vi "Sweep Set.vi"(8 "error in (no error)":errorcluster, 9 "Sweep outfile":path, 10 "addr":i32, 11 "instrument handle":refnum<k15>) -> (0 "error out":errorcluster, 1 "final current (A)":dbl, 2 "final resistance (ohm)":dbl, 3 "instrument handle out":refnum<k15>)   [LabVIEW 2018]
uses:
  <vilib>/Utility/file.llb/Write Delimited Spreadsheet (DBL).vi
panel:
  out "i":i32
  out "PW":i32
  out "BL voltage (V)":dbl
  out "WL voltage (V)":dbl
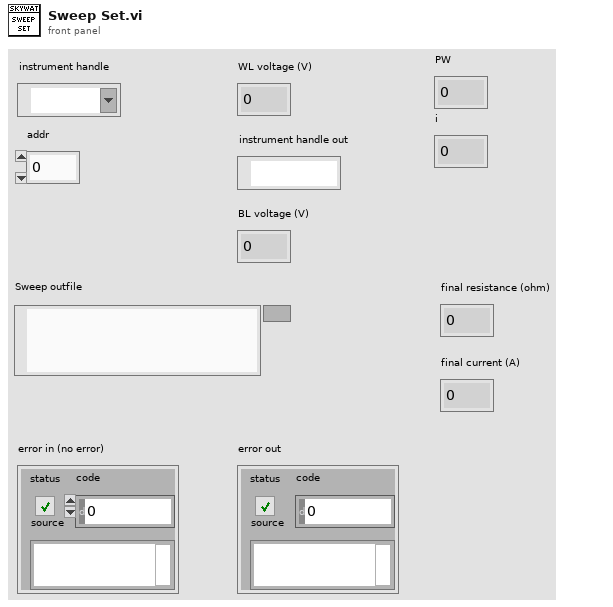
[diagram p1: front panel]
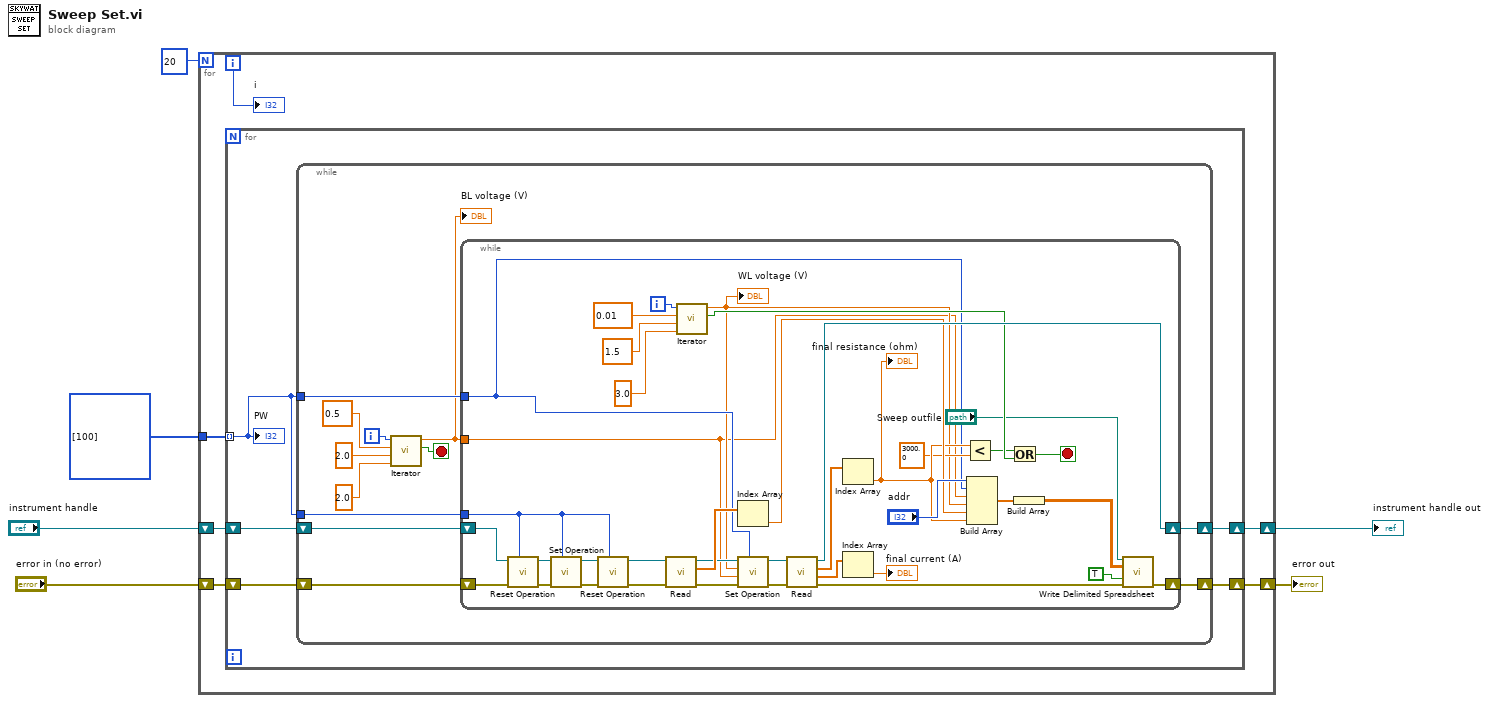
[diagram p0: block diagram]
diagram:
  n1 = for {
    N: 20 -> [_]
    tunnel: i32[] [100] -> [w8]
    shift-right: [w12] -> w6
    shift-left: "instrument handle" -> [w11]
    shift-right: [w9] -> w3
    shift-left: "error in (no error)" -> [w10]
    i -> [w7]
    n2 = for {
      shift-right: [w17] -> w12
      shift-left: w11 -> [w16]
      shift-right: [w14] -> w9
      shift-left: w10 -> [w15]
      tunnel: w8 -> [w13] mode=indexing
      n3 = while {
        shift-right: [w26] -> w17
        shift-left: w16 -> [w19]
        shift-right: [w25] -> w14
        shift-left: w15 -> [w18]
        tunnel: w13 -> [w23]
        tunnel: w13 -> [w20]
        i -> [w27]
        stop <- w22 stop-if-true
        n4 = call "Iterator.vi"("Final Value"=2.0 ("y"), "Initial Value"=2.0 ("y"), "Step"=0.5 ("x"), "i"=w27) -> ("End Loop"=w22:bool, "Current Value"=w21:dbl)  [unwired: 6 in]
        "BL voltage (V)" <- w21
        n5 = while {
          shift-right: [w57] -> w26
          shift-left: w19 -> [w37]
          shift-right: [w60] -> w25
          shift-left: w18 -> [w34]
          tunnel: w21 -> [w39]
          tunnel: w23 -> [w42]
          tunnel: w20 -> [w38]
          i -> [w67]
          stop <- w51 stop-if-true
          n6 = call "Reset Operation.vi"("PW"=w38, "error in (no error)"=w34, "instrument handle"=w37) -> ("error out"=w33:errorcluster, "instrument handle out"=w32:refnum<k15>)  [unwired: 7 in]
          n7 = call "Set Operation.vi"("PW"=w38, "error in (no error)"=w33, "instrument handle"=w32) -> ("error out"=w31:errorcluster, "instrument handle out"=w30:refnum<k15>)  [unwired: 7 in]
          n8 = call "Reset Operation.vi"("PW"=w38, "error in (no error)"=w31, "instrument handle"=w30) -> ("error out"=w35:errorcluster, "instrument handle out"=w36:refnum<k15>)  [unwired: 7 in]
          n9 = call "Read.vi"("error in (no error)"=w35, "instrument handle"=w36) -> ("error out"=w45:errorcluster, "resistances (ohm)"=w53:dbl[], "instrument handle out"=w46:refnum<k15>)  [unwired: 6 in, 1 out]
          n10 = call "Iterator.vi"("Final Value"=3.0 ("y"), "Initial Value"=1.5 ("y"), "Step"=0.01 ("x"), "i"=w67) -> ("End Loop"=w50:bool, "Current Value"=w40:dbl)  [unwired: 6 in]
          "WL voltage (V)" <- w40
          n11 = Index Array(array=w53) -> (element=w52:dbl)  [unwired: 1 in]
          n12 = call "Set Operation.vi"("PW"=w42, "error in (no error)"=w45, "BLV"=w39, "WLV"=w40, "instrument handle"=w46) -> ("error out"=w44:errorcluster, "instrument handle out"=w43:refnum<k15>)  [unwired: 5 in]
          n13 = call "Read.vi"("error in (no error)"=w44, "instrument handle"=w43) -> ("error out"=w58:errorcluster, "currents (A)"=w55:dbl[], "resistances (ohm)"=w56:dbl[], "instrument handle out"=w57:refnum<k15>)  [unwired: 6 in]
          n14 = Index Array(array=w56) -> (element=w49:dbl)  [unwired: 1 in]
          "final resistance (ohm)" <- w49
          n15 = Index Array(array=w55) -> (element=→"final current (A)":dbl)  [unwired: 1 in]
          n16 = Less?(x=w49, y=3000.0 ("x")) -> (x < y?=w47:bool)
          n17 = Build Array("addr", w42, w39, w40, w52, w49) -> (w62:dbl[])
          n18 = Or(x=w47, y=w50) -> (x .or. y?=w51:bool)
          n19 = Build Array(w62) -> (w63:dbl[][])
          n20 = call-poly <vilib>:"Write Delimited Spreadsheet.vi"("file path (dialog if empty)"="Sweep outfile", "2D data"=w63, "append to file? (new file:F)"=TRUE, "error in (no error)"=w58) -> ("error out"=w60:errorcluster)  [unwired: 10 in, 1 out]
        }
      }
      "PW" <- w13
    }
    "i" <- w7
  }
  "error out" <- w3
  "instrument handle out" <- w6
